vi "Do data taking procedure (SubVI).vi"(0 "input cluster":T1, 1 "duration data taking (s)":i32, 2 "queue in":refnum<queue>, 3 "error in (no error)":errorcluster, 4 "filament warmup duration (s)":i32) -> (6 "error out":errorcluster)   [LabVIEW 2016]
panel:
  out "has completed procedure?":bool=TRUE
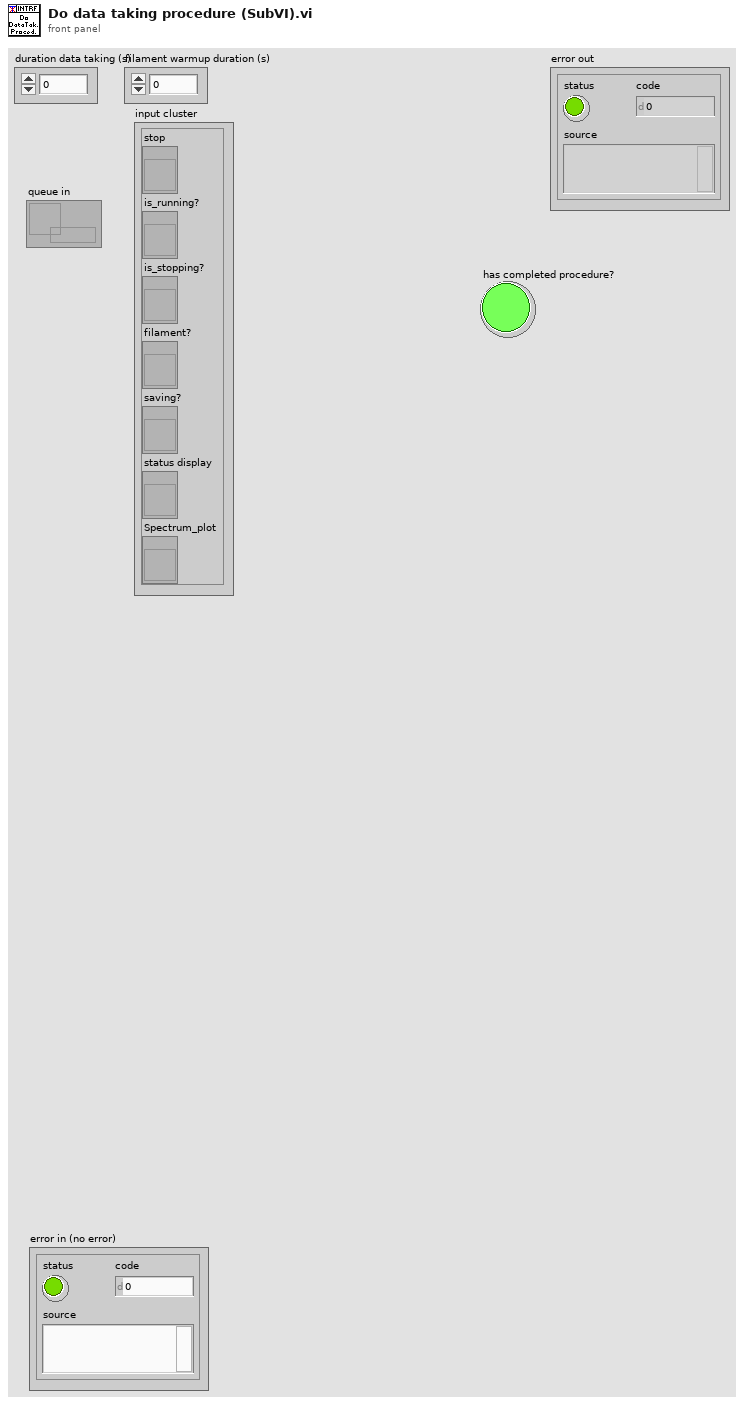
[diagram p1: front panel]
types:
  T1 = cluster{"stop":refnum<vi>, "is_running?":refnum<vi>, "is_stopping?":refnum<vi>, "filament?":refnum<vi>, "saving?":refnum<vi>, "status display":refnum<vi>, "Spectrum_plot":refnum<vi>}
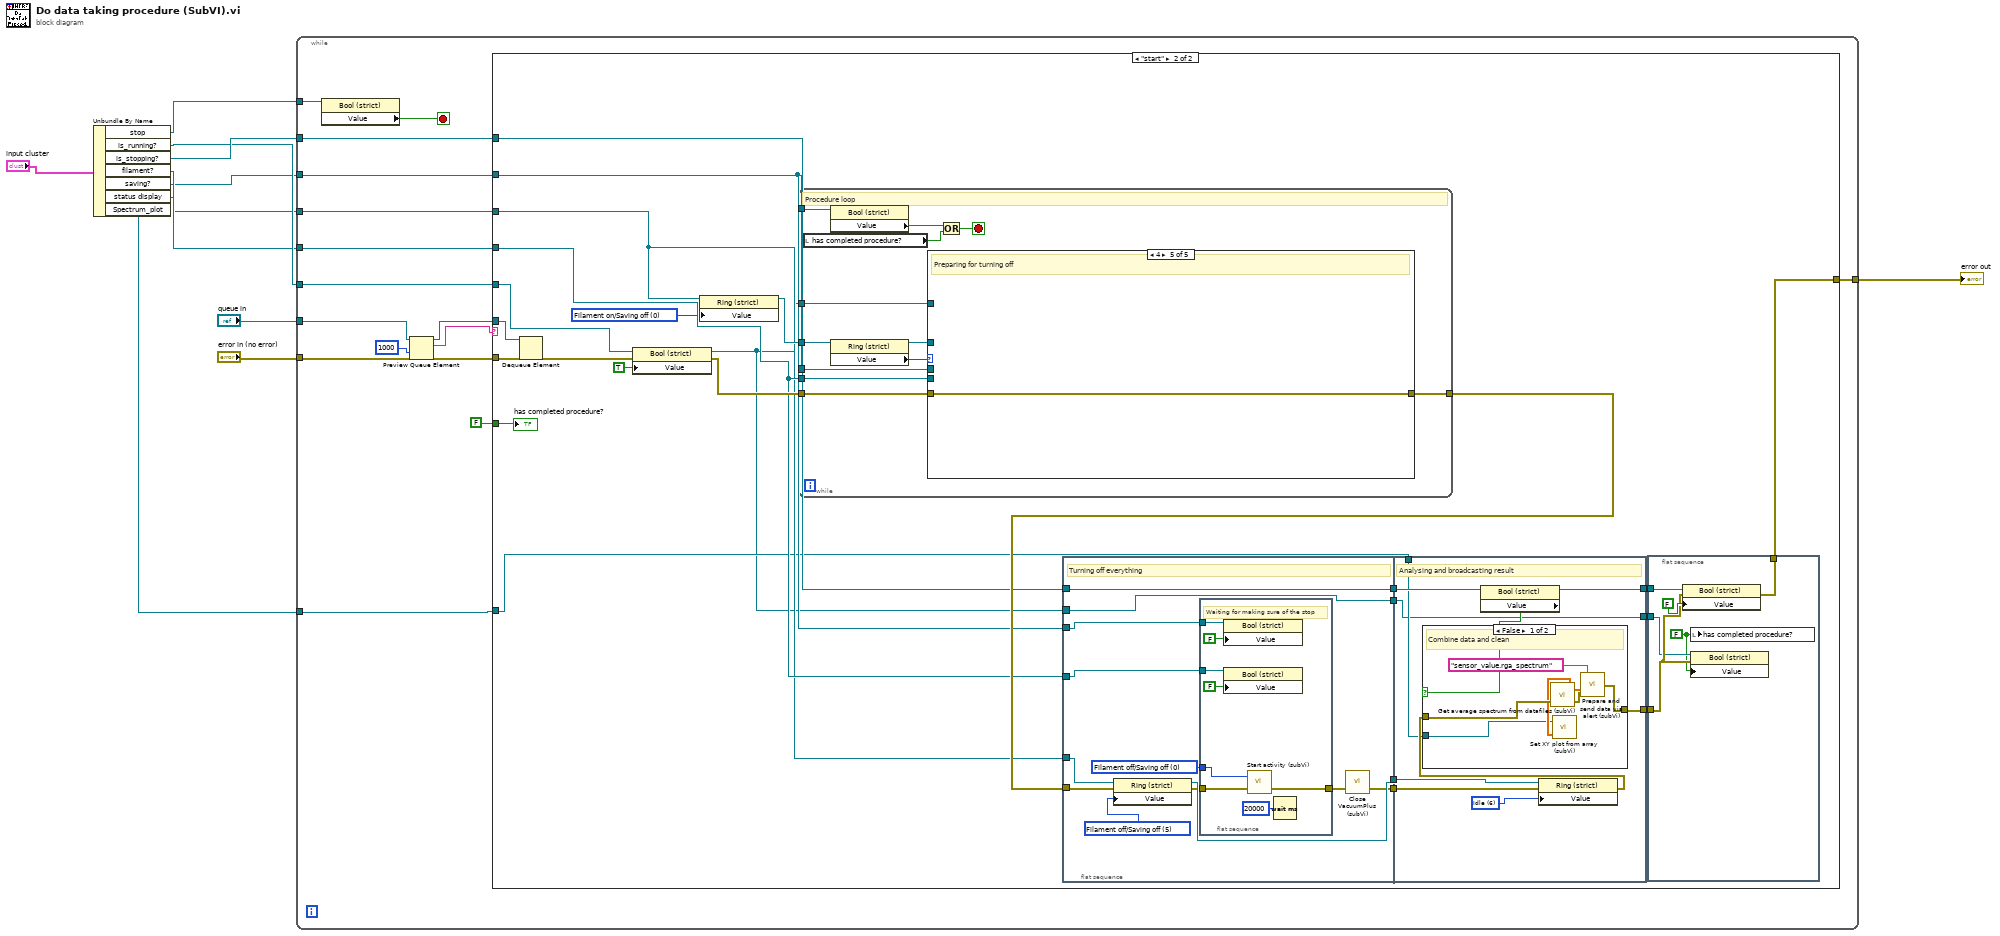
[diagram p0: block diagram]
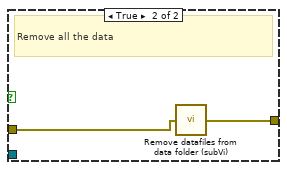
[diagram p3: hidden frame]
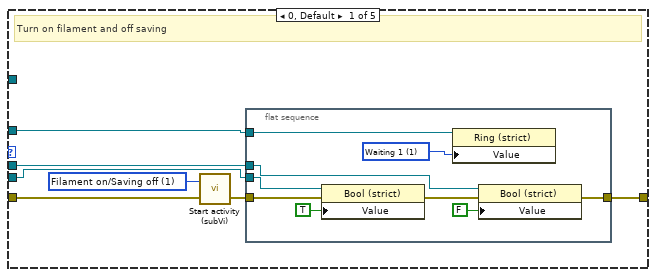
[diagram p4: hidden frame]
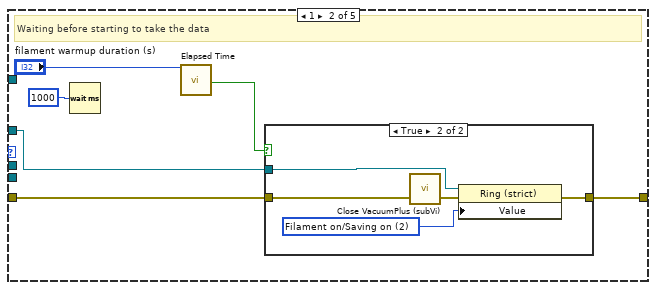
[diagram p5: hidden frame]
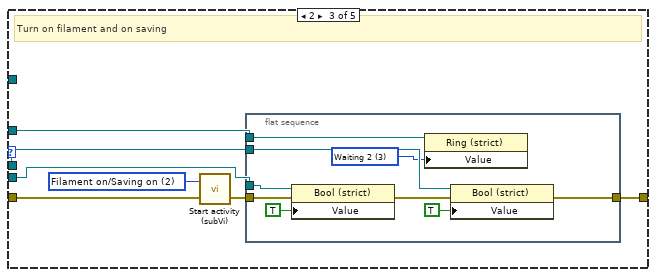
[diagram p7: hidden frame]
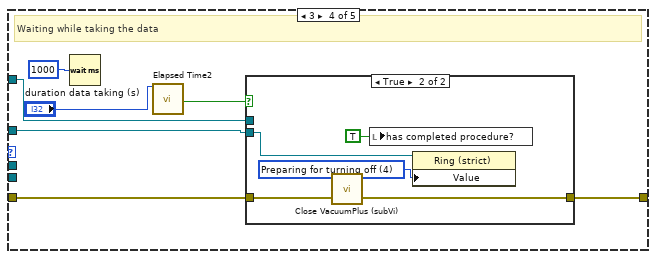
[diagram p8: hidden frame]
diagram:
  n1 = Unbundle By Name("input cluster") -> ("stop"=w8:refnum<vi>, "is_running?"=w6:refnum<vi>, "is_stopping?"=w7:refnum<vi>, "filament?"=w5:refnum<vi>, "saving?"=w4:refnum<vi>, "status display"=w3:refnum<vi>, "Spectrum_plot"=w1:refnum<vi>)
  n2 = while {
    tunnel: "queue in" -> [w27]
    tunnel: "error in (no error)" -> [w25]
    tunnel: w8 -> [w20]
    tunnel: w7 -> [w19]
    tunnel: w3 -> [w18]
    tunnel: w5 -> [w15]
    tunnel: w4 -> [w17]
    tunnel: w6 -> [w16]
    tunnel: [w14] -> w9
    tunnel: w1 -> [w13]
    stop <- w26 stop-if-true
    n3 = property class="Bool (strict)"(reference=w20) -> ("Value"=w26:bool)  [unwired: 1 in, 2 out]
    n4 = Preview Queue Element(queue=w27, timeout in ms (-1)=1000, error in (no error)=w25) -> (queue out=w21:refnum<queue>, element=w23:string, error out=w22:errorcluster)  [unwired: 1 out]
    n5 = case shown="\"start\"" w23 {
      tunnel: w22 -> [w28 w50]
      tunnel: w21 -> [_ w51]
      tunnel: w19 -> [_ w46]
      tunnel: w18 -> [_ w40]
      tunnel: w17 -> [_ w41]
      tunnel: w16 -> [_ w44]
      tunnel: w15 -> [_ w45]
      tunnel: [w28 w36] -> w14
      tunnel: w13 -> [_ w35]
      tunnel: FALSE ("has completed procedure?") -> [_ w30]
      frame "", Default {
      }
      frame "start" {
        w29 = u16 0 items=["Filament on/Saving off", "Waiting 1", "Filament on/Saving on", "Waiting 2", "Preparing for turning off", "Filament off/Saving off", "Idle"] ("status display")
        n6 = Dequeue Element(queue=w51, error in (no error)=w50) -> (error out=w48:errorcluster)  [unwired: 1 in, 3 out]
        n7 = property class="Bool (strict)"(reference=w44, error in=w48, "Value"=TRUE) -> (reference out=w33:refnum<vi>, error out=w47:errorcluster)
        n8 = property class="Ring (strict)"(reference=w40, "Value"=w29) -> (reference out=w43:refnum<vi>)  [unwired: 1 in, 1 out]
        n9 = while {
          tunnel: w47 -> [w107]
          tunnel: [w104] -> w52
          tunnel: w43 -> [w103]
          tunnel: w33 -> [w98]
          tunnel: w46 -> [w102]
          tunnel: w45 -> [w101]
          tunnel: w41 -> [w100]
          stop <- w105 stop-if-true
          # "Procedure loop"
          n10 = local read "has completed procedure?"() -> (w97:bool)
          n11 = property class="Bool (strict)"(reference=w102) -> ("Value"=w106:bool)  [unwired: 1 in, 2 out]
          n12 = property class="Ring (strict)"(reference=w103) -> (reference out=w99:refnum<vi>, "Value"=w108:u16)  [unwired: 1 in, 1 out]
          n13 = case shown="4" w108 {
            tunnel: w107 -> [w114 w128 w142 w157 w166]
            tunnel: [w112 w127 w140 w156 w166] -> w104
            tunnel: w98 -> [_ _ _ w154 _]
            tunnel: w101 -> [w110 _ w138 _ _]
            tunnel: w100 -> [w109 _ w137 _ _]
            tunnel: w99 -> [w111 w125 w139 w153 _]
            frame 0, Default {
              w115 = u16 1 items=["Filament off/Saving off", "Filament on/Saving off", "Filament on/Saving on"] ("Text Ring")
              # "Turn on filament and off saving"
              n14 = call "Start activity (subVi).vi"("error in"=w114, "Text Ring"=w115) -> ("error out"=w113:errorcluster)  [unwired: 1 in]
              n15 = flat-sequence {
                tunnel: w113 -> [w123]
                tunnel: [w120] -> w112
                tunnel: w111 -> [w119]
                tunnel: w110 -> [w118]
                tunnel: w109 -> [w117]
                frame #0 {
                  w116 = u16 1 items=["Filament on/Saving off", "Waiting 1", "Filament on/Saving on", "Waiting 2", "Preparing for turning off", "Filament off/Saving off", "Idle"] ("status display")
                  n16 = property class="Bool (strict)"(reference=w118, error in=w123, "Value"=TRUE) -> (error out=w121:errorcluster)  [unwired: 1 out]
                  n17 = property class="Ring (strict)"(reference=w119, "Value"=w116) -> ()  [unwired: 1 in, 2 out]
                  n18 = property class="Bool (strict)"(reference=w117, error in=w121, "Value"=FALSE) -> (error out=w120:errorcluster)  [unwired: 1 out]
                }
              }
            }
            frame 1 {
              # "Waiting before starting to take the data"
              n19 = Wait (ms)(milliseconds to wait=u32 1000) -> ()  [unwired: 1 out]
              n20 = call "Elapsed Time"("Time Target (s)"="filament warmup duration (s)") -> ("Time has Elapsed"=w129:bool)  [unwired: 11 in, 7 out]
              n21 = case shown="True" w129 {
                tunnel: w128 -> [w131 w136]
                tunnel: [w131 w133] -> w127
                tunnel: w125 -> [_ w135]
                frame False {
                }
                frame True {
                  w132 = u16 2 items=["Filament on/Saving off", "Waiting 1", "Filament on/Saving on", "Waiting 2", "Preparing for turning off", "Filament off/Saving off", "Idle"] ("status display")
                  n22 = call "Close VacuumPlus (subVi).vi"("error in (no error)"=w136) -> ("error out"=w134:errorcluster)  [unwired: 1 in, 1 out]
                  n23 = property class="Ring (strict)"(reference=w135, error in=w134, "Value"=w132) -> (error out=w133:errorcluster)  [unwired: 1 out]
                }
              }
            }
            frame 2 {
              w143 = u16 2 items=["Filament off/Saving off", "Filament on/Saving off", "Filament on/Saving on"] ("Text Ring")
              # "Turn on filament and on saving"
              n24 = call "Start activity (subVi).vi"("error in"=w142, "Text Ring"=w143) -> ("error out"=w141:errorcluster)  [unwired: 1 in]
              n25 = flat-sequence {
                tunnel: w141 -> [w151]
                tunnel: [w145] -> w140
                tunnel: w139 -> [w148]
                tunnel: w138 -> [w147]
                tunnel: w137 -> [w146]
                frame #0 {
                  w144 = u16 3 items=["Filament on/Saving off", "Waiting 1", "Filament on/Saving on", "Waiting 2", "Preparing for turning off", "Filament off/Saving off", "Idle"] ("status display")
                  n26 = property class="Bool (strict)"(reference=w147, error in=w151, "Value"=TRUE) -> (error out=w149:errorcluster)  [unwired: 1 out]
                  n27 = property class="Ring (strict)"(reference=w148, "Value"=w144) -> ()  [unwired: 1 in, 2 out]
                  n28 = property class="Bool (strict)"(reference=w146, error in=w149, "Value"=TRUE) -> (error out=w145:errorcluster)  [unwired: 1 out]
                }
              }
            }
            frame 3 {
              # "Waiting while taking the data"
              n29 = Wait (ms)(milliseconds to wait=u32 1000) -> ()  [unwired: 1 out]
              n30 = call "Elapsed Time2"("Time Target (s)"="duration data taking (s)") -> ("Time has Elapsed"=w158:bool)  [unwired: 11 in, 7 out]
              n31 = case shown="True" w158 {
                tunnel: w157 -> [w160 w165]
                tunnel: [w160 w164] -> w156
                tunnel: w154 -> [_ _]
                tunnel: w153 -> [_ w162]
                frame False {
                }
                frame True {
                  w161 = u16 4 items=["Filament on/Saving off", "Waiting 1", "Filament on/Saving on", "Waiting 2", "Preparing for turning off", "Filament off/Saving off", "Idle"] ("status display")
                  n32 = call "Close VacuumPlus (subVi).vi"("error in (no error)"=w165) -> ("error out"=w164:errorcluster)  [unwired: 1 in, 1 out]
                  n33 = local write "has completed procedure?"(TRUE ("has completed procedure?")) -> ()
                  n34 = property class="Ring (strict)"(reference=w162, "Value"=w161) -> ()  [unwired: 1 in, 2 out]
                }
              }
            }
            frame 4 {
              # "Preparing for turning off"
            }
          }
          n35 = Or(x=w106, y=w97) -> (x .or. y?=w105:bool)
        }
        n36 = flat-sequence {
          tunnel: w52 -> [w66]
          tunnel: w40 -> [w69]
          tunnel: w41 -> [w62]
          tunnel: w46 -> [w63]
          tunnel: w45 -> [w61]
          tunnel: [w68] -> w42
          tunnel: [w65] -> w39
          tunnel: [w63] -> w37
          tunnel: w33 -> [w60]
          tunnel: [w60] -> w32
          tunnel: w42 -> [w88]
          tunnel: w39 -> [w87]
          tunnel: [w85] -> w38
          tunnel: w37 -> [w86]
          tunnel: [w82] -> w34
          tunnel: w35 -> [w81]
          tunnel: w32 -> [w80]
          tunnel: [w80] -> w31
          frame #0 {
            w59 = u16 5 items=["Filament on/Saving off", "Waiting 1", "Filament on/Saving on", "Waiting 2", "Preparing for turning off", "Filament off/Saving off", "Idle"] ("status display")
            w67 = u16 0 items=["Filament off/Saving off", "Filament on/Saving off", "Filament on/Saving on"] ("Text Ring")
            # "Turning off everything"
            n37 = property class="Ring (strict)"(reference=w69, error in=w66, "Value"=w59) -> (reference out=w68:refnum<vi>, error out=w64:errorcluster)
            n38 = flat-sequence {
              tunnel: [w78] -> w70
              tunnel: w67 -> [w77]
              tunnel: w64 -> [w76]
              tunnel: w62 -> [w72]
              tunnel: w61 -> [w71]
              frame #0 {
                # "Waiting for making sure of the stop"
                n39 = property class="Bool (strict)"(reference=w72, "Value"=FALSE) -> ()  [unwired: 1 in, 2 out]
                n40 = property class="Bool (strict)"(reference=w71, "Value"=FALSE) -> ()  [unwired: 1 in, 2 out]
                n41 = call "Start activity (subVi).vi"("error in"=w76, "Text Ring"=w77) -> ("error out"=w78:errorcluster)  [unwired: 1 in]
                n42 = Wait (ms)(milliseconds to wait=u32 20000) -> ()  [unwired: 1 out]
              }
            }
            n43 = call "Close VacuumPlus (subVi).vi"("error in (no error)"=w70) -> ("error out"=w65:errorcluster)  [unwired: 1 in, 1 out]
          }
          frame #1 {
            w79 = u16 6 items=["Filament on/Saving off", "Waiting 1", "Filament on/Saving on", "Waiting 2", "Preparing for turning off", "Filament off/Saving off", "Idle"] ("status display")
            # "Analysing and broadcasting result"
            n44 = property class="Bool (strict)"(reference=w86) -> (reference out=w85:refnum<vi>, "Value"=w84:bool)  [unwired: 1 in, 1 out]
            n45 = property class="Ring (strict)"(reference=w88, error in=w87, "Value"=w79) -> (error out=w83:errorcluster)  [unwired: 1 out]
            n46 = case shown="False" w84 {
              tunnel: w83 -> [w94 w96]
              tunnel: [w92 w95] -> w82
              tunnel: w81 -> [w89 _]
              frame False {
                # "Combine data and clean"
                n47 = call "Get average spectrum from datafiles (subVi).vi"("error in"=w94) -> ("error out"=w93:errorcluster, "Average array"=w90:dbl[][])  [unwired: 1 in]
                n48 = call "Set XY plot from array (subVi).vi"("Average array"=w90, "Spectrum_plot"=w89) -> ()  [unwired: 1 in, 1 out]
                n49 = call "Prepare and send data via alert (subVi).vi"("error in (no error)"=w93, "Average array"=w90, "target"="sensor_value.rga_spectrum") -> ("error out"=w92:errorcluster)
              }
              frame True {
                # "Remove all the data"
                n50 = call "Remove datafiles from data folder (subVi).vi"("error in"=w96) -> ("error out"=w95:errorcluster)
              }
            }
          }
        }
        n51 = flat-sequence {
          tunnel: w38 -> [w57]
          tunnel: [w56] -> w36
          tunnel: w34 -> [w55]
          tunnel: w31 -> [w54]
          frame #0 {
            w53 = FALSE ("Value")
            n52 = property class="Bool (strict)"(reference=w57, error in=w55, "Value"=FALSE) -> (error out=w56:errorcluster)  [unwired: 1 out]
            n53 = local write "has completed procedure?"(w53) -> ()
            n54 = property class="Bool (strict)"(reference=w54, error in=w55, "Value"=w53) -> ()  [unwired: 2 out]
          }
        }
        "has completed procedure?" <- w30
      }
    }
  }
  "error out" <- w9
